vi "Evaluate Guess.vi"(8 "error in":errorcluster, 10 "Guess":string, 11 "Current Word":string) -> (0 "error out":errorcluster, 3 "Result":string)   [LabVIEW 2020, in "Wordle Engine.lvlib"]
uses:
  Wordle Engine.lvlib
  <vilib>/Utility/error.llb/Error Cluster From Error Code.vi
  <vilib>/ErrorRing/Error Ring.xnode
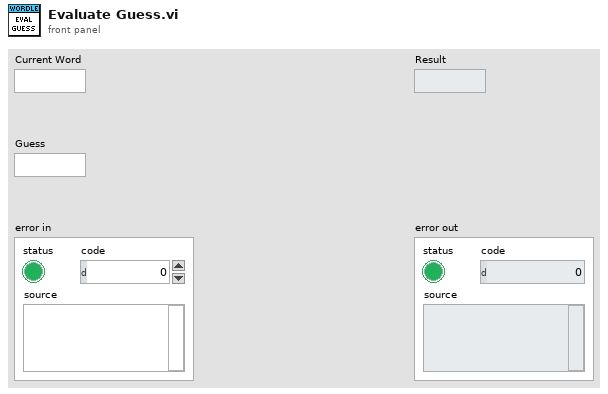
[diagram p1: front panel]
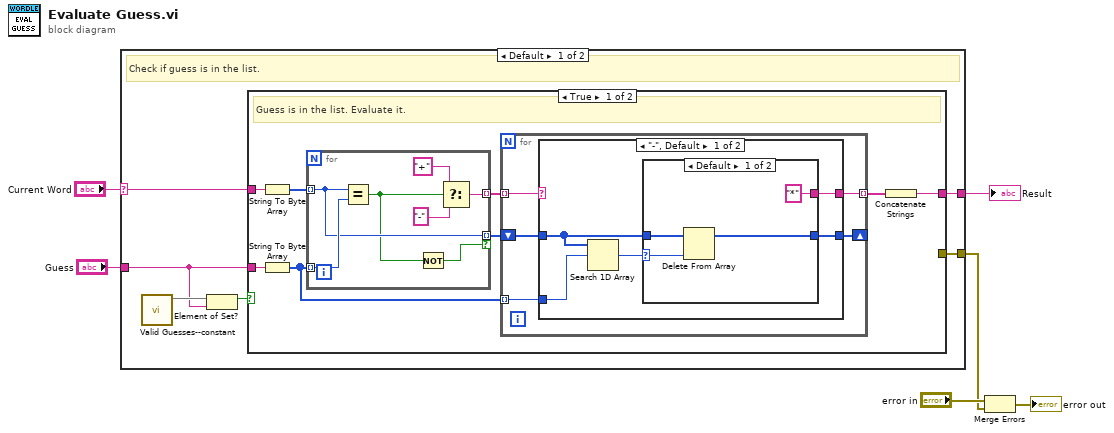
[diagram p0: block diagram]
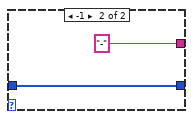
[diagram p2: hidden frame]
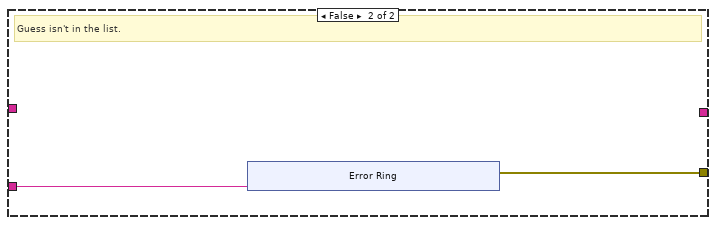
[diagram p4: hidden frame]
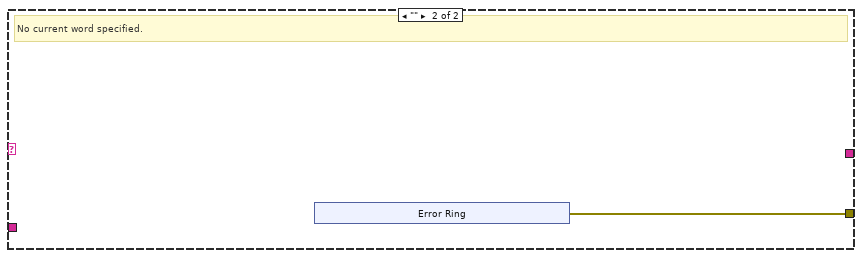
[diagram p5: hidden frame]
diagram:
  n1 = case shown="Default" "Current Word" {
    selector: "Current Word" -> [w11 _]
    tunnel: [w12 w55] -> w3
    tunnel: "Guess" -> [w8 _]
    tunnel: [w10 _] -> w1
    frame Default {
      # "Check if guess is in the list."
      n2 = call "Valid Guesses--constant.vi"() -> ("Valid Guesses"=w9:set{string})  [unwired: 11 in]
      n3 = Element of Set?(10:w8, 11:w9) -> (3:w7:bool)
      n4 = case shown="True" w7 {
        tunnel: [_ w47] -> w12
        tunnel: w8 -> [w19 w46]
        tunnel: w11 -> [w20 _]
        tunnel: [w15 _] -> w10
        frame True {
          # "Guess is in the list. Evaluate it."
          n5 = String To Byte Array(string=w20) -> (unsigned byte array=w14:u8[])
          n6 = String To Byte Array(string=w19) -> (unsigned byte array=w17:u8[])
          n7 = for {
            tunnel: w14 -> [w23] mode=indexing
            tunnel: w17 -> [w27] mode=indexing
            tunnel: [w24] -> w18 mode=indexing
            tunnel: [w23] -> w13 mode=indexing if=w21
            n8 = Equal?(x=w23, y=w27) -> (x = y?=w22:bool)
            n9 = Not(x=w22) -> (.not. x?=w21:bool)
            n10 = Select(t="+", s=w22, f="-") -> (s? t:f=w24:string)
          }
          n11 = for {
            tunnel: w18 -> [w32] mode=indexing
            tunnel: w17 -> [w29] mode=indexing
            tunnel: [w31] -> w16 mode=indexing
            shift-right: [w28] -> _
            shift-left: w13 -> [w30]
            n12 = case shown="\"-\", Default" w32 {
              selector: w32 -> [_ w45]
              tunnel: [w35 w45] -> w31
              tunnel: w30 -> [w33 w44]
              tunnel: w29 -> [w37 _]
              tunnel: [w34 w44] -> w28
              frame "-", Default {
                n13 = Search 1D Array(1D array=w33, element=w37) -> (index of element=w36:i32)  [unwired: 1 in]
                n14 = case shown="Default" w36 {
                  selector: w36 -> [w40 _]
                  tunnel: ["*" "-"] -> w35
                  tunnel: [w39 w42] -> w34
                  tunnel: w33 -> [w41 w42]
                  frame Default {
                    n15 = Delete From Array(array=w41, index=w40) -> (array with subset deleted=w39:u8[])  [unwired: 1 in, 1 out]
                  }
                  frame -1 {
                  }
                }
              }
              frame "+" {
              }
            }
          }
          n16 = Concatenate Strings(w16) -> (w15:string)
        }
        frame False {
          # "Guess isn't in the list."
          n17 = xnode "Error Ring"("parameter 0"=w46) -> ("error out"=w47:errorcluster)
        }
      }
    }
    frame "" {
      # "No current word specified."
      n18 = xnode "Error Ring"() -> ("error out"=w55:errorcluster)
    }
  }
  "Result" <- w1
  n19 = Merge Errors("error in", w3) -> (→"error out":errorcluster)
